vi "getWaypoints.vi"(11 "PassBouy.lvclass in":refnum<class "PassBouy.lvclass">) -> (2 "Array":refnum<class "Waypoint.lvclass">[](array[class]), 3 "PassBouy.lvclass out":refnum<class "PassBouy.lvclass">)   [LabVIEW 2012, in "PassBouy.lvclass"]
doc: "Takes a bouy object. Returns an array of waypoints nessesary for going through the given set of bouys. In it's current form these bouys form a line perpendicular to the line formed by the two bouys.\n\n2/5/2014\nMac-I Crowell"
uses:
  PassBouy.lvclass
  Waypoint/Waypoint.lvclass
panel:
  out "Error Out":errorcluster
  in  "Error In":errorcluster
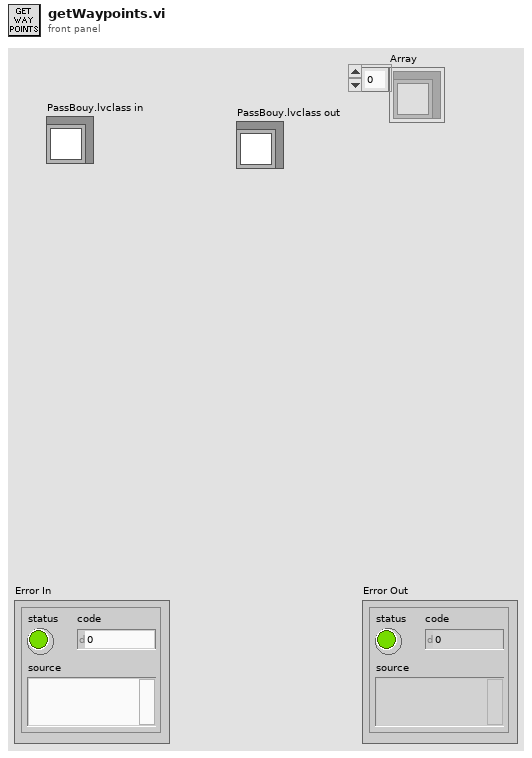
[diagram p1: front panel]
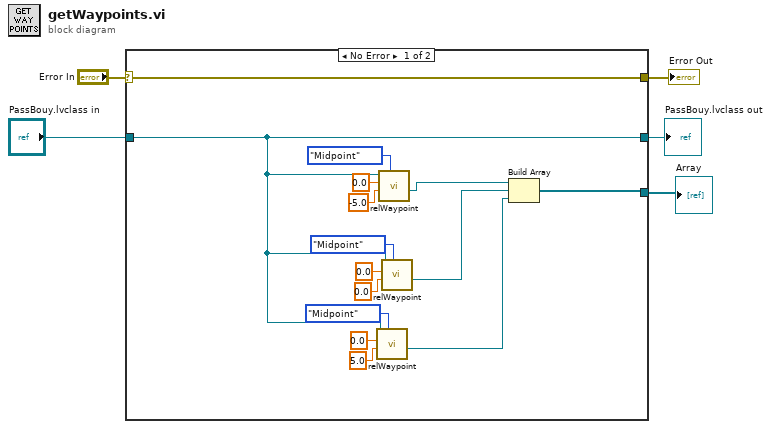
[diagram p0: block diagram]
diagram:
  n1 = case shown="No Error" "Error In" {
    selector: "Error In" -> [w20 w21]
    tunnel: [w20 w21] -> w4
    tunnel: "PassBouy.lvclass in" -> [w6 w22]
    tunnel: [w6 w22] -> w3
    tunnel: [w18 _] -> w1
    frame No Error {
      n2 = call "relWaypoint.vi"("Base Point"=enum16{"Port", "Midpoint", "Starboard"}."Midpoint", "Y coord"=5.0 ("X coord"), "X coord"=0.0, "PassBouy.lvclass"=w6) -> ("Waypoint Out"=w8:refnum<class "Waypoint.lvclass">)  [unwired: 5 in, 2 out]
      n3 = call "relWaypoint.vi"("Base Point"=enum16{"Port", "Midpoint", "Starboard"}."Midpoint", "Y coord"=-5.0 ("X coord"), "X coord"=0.0, "PassBouy.lvclass"=w6) -> ("Waypoint Out"=w17:refnum<class "Waypoint.lvclass">)  [unwired: 5 in, 2 out]
      n4 = call "relWaypoint.vi"("Base Point"=enum16{"Port", "Midpoint", "Starboard"}."Midpoint", "Y coord"=0.0 ("X coord"), "X coord"=0.0, "PassBouy.lvclass"=w6) -> ("Waypoint Out"=w7:refnum<class "Waypoint.lvclass">)  [unwired: 5 in, 2 out]
      n5 = Build Array(w17, w7, w8) -> (w18:refnum<class "Waypoint.lvclass">[])
    }
    frame Error {
    }
  }
  "Error Out" <- w4
  "PassBouy.lvclass out" <- w3
  "Array" <- w1
